vi "6XNN.vi"(11 "Variables and Memory in":T1 {"GFX" format="%02x"}) -> (3 "Variables and Memory out":T1 {"GFX" format="%02x"})   [LabVIEW 2021]
uses:
  Controls/ClusterF.ctl
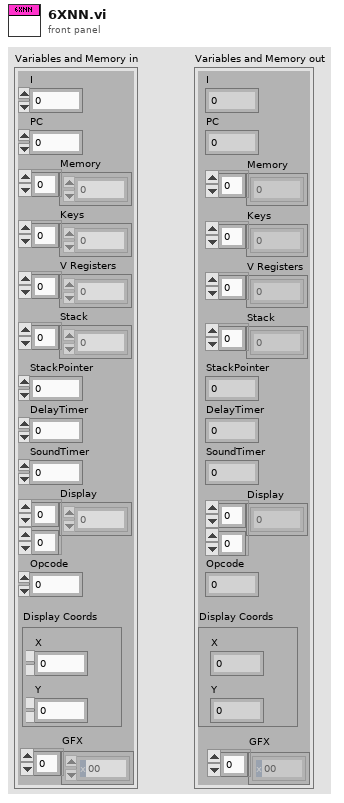
[diagram p1: front panel]
types:
  T1 = typedef "ClusterF.ctl" = cluster{"I":u16, "PC":u16, "Memory":u8[], "Keys":u8[], "V Registers":u8[], "Stack":u16[], "StackPointer":u16, "DelayTimer":u8, "SoundTimer":u8, "Display":u8[][], "Opcode":u16, "Display Coords":cluster{"X":u8, "Y":u8}, "GFX":u8[]}
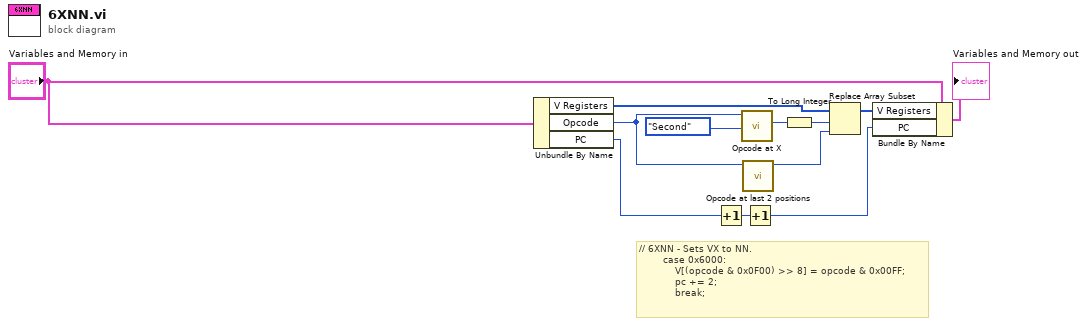
[diagram p0: block diagram]
diagram:
  # "// 6XNN - Sets VX to NN.\n        case 0x6000:\n            V[(opcode & 0x0F00) >> 8] = opcode & 0x00FF;\n            pc += 2;\n            break;"
  n1 = Unbundle By Name("Variables and Memory in") -> ("V Registers"=w12:u8[], "Opcode"=w10:u16, "PC"=w4:u16)
  n2 = Increment(x=w4) -> (x+1=w5:u16)
  n3 = call "Opcode at X.vi"("X Position"=enum16{"First", "Second", "Third", "Fourth"}."Second", "Opcode"=w10) -> ("Opcode at X Position (U8)"=w9:u8)  [unwired: 9 in]
  n4 = call "Opcode at last 2 positions.vi"("Opcode"=w10) -> ("00FF"=w11:u8)  [unwired: 10 in]
  n5 = Increment(x=w5) -> (x+1=w6:u16)
  n6 = To Long Integer(number=w9) -> (32bit integer=w7:i32)
  n7 = Replace Array Subset(array=w12, new element=w11, index=w7) -> (w3:u8[])
  n8 = Bundle By Name(cluster="Variables and Memory in", "V Registers"=w3, "PC"=w6) -> (→"Variables and Memory out":T1)
